vi "SVPO Power in Band.vi"   [LabVIEW 2017]
doc: "Computes the aggregate power of a linear-scale power spectrum within the specified frequency <B>range</B> of the input spectrum. Use this VI on embedded targets that have limited computational resources. Wire data to the <B>spectrum [EU^2 rms]</B> input to determine the polymorphic instance to use or manually select the instance."
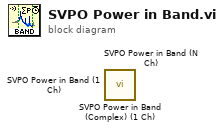
[diagram p0: block diagram]
diagram:
  n1 = call <vilib>:"SVPO Power in Band (Complex) (1 Ch).vi"() -> ()  [unwired: 19 in, 1 out]
  n2 = call <vilib>:"SVPO Power in Band (N Ch).vi"() -> ()  [unwired: 19 in, 1 out]
  n3 = call <vilib>:"SVPO Power in Band (1 Ch).vi"() -> ()  [unwired: 19 in, 1 out]
